vi "cos circle.vi"() -> (3 "cos(x)":dbl[](array[numeric]))   [LabVIEW 2014]
panel:
  out "Waveform Graph":dbl[](graph)
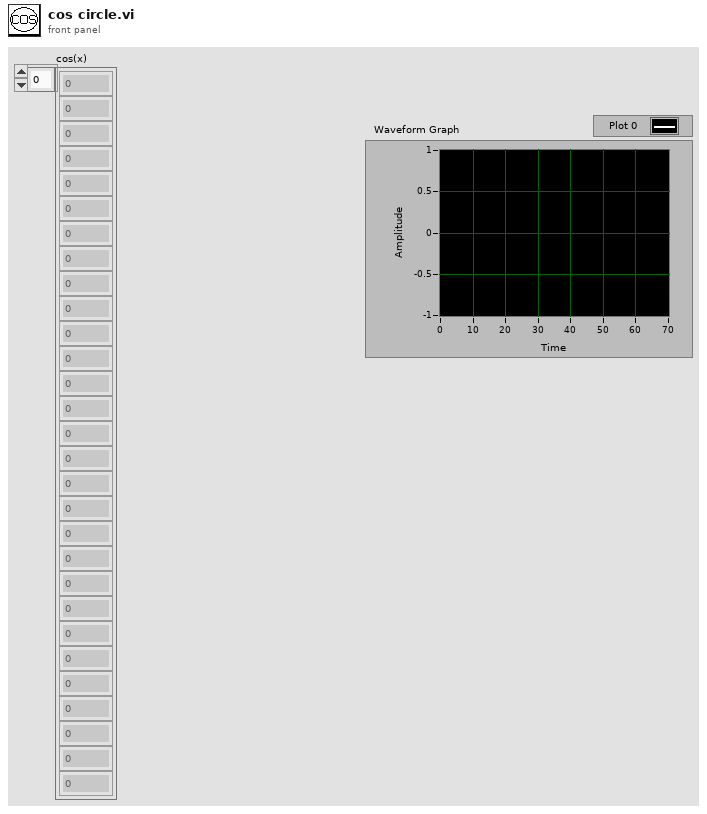
[diagram p1: front panel]
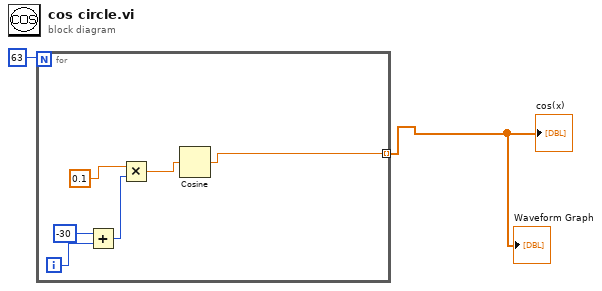
[diagram p0: block diagram]
diagram:
  n1 = for {
    N: 63 -> [_]
    tunnel: [w8] -> w1 mode=indexing
    i -> [w5]
    n2 = Add(x=-30, y=w5) -> (x+y=w3:i32)
    n3 = Multiply(x=0.1, y=w3) -> (x*y=w7:dbl)
    n4 = Cosine(x=w7) -> (cos(x)=w8:dbl)
  }
  "cos(x)" <- w1
  "Waveform Graph" <- w1
